vi "File handling.vi"(1 "Loop ID":u16, 11 "error out":errorcluster) -> ()   [LabVIEW 2011]
uses:
  Status Digitalish.ctl
  emi Lib/System 01/0 - General/App/Loop control 2/Private/_emi_ SMLoop start condition.vi
  emi Lib/System 01/0 - General/App/Loop control 2/Private/_emi_ SMLoop Error Check.vi
  emi Lib/Basic/0 - General/Error/emi_Is Error.vi
  emi Lib/System 01/0 - General/App/Loop control 2/Private/_emi_SMLoop Register new.vi
  emi Lib/System 01/0 - General/S&E reporting/emi_Send S&E Error message.vi
  emi Lib/Basic/0 - General/Error/emi_ Is Error state.vi
  emi Lib/System 01/0 - General/emi_Read System ID.vi
  emi Lib/System 01/0 - General/App/Loop control/Private/_emi_GFV Loop Linking.vi
  emi Lib/System 01/0 - General/App/Loop control/Private/_emi_GFV Loop Enable.vi
  emi Lib/System 01/0 - General/App/Loop control 2/Private/_emi_ SMLoop Restart.vi
  emi Lib/System 01/0 - General/App/Private/_emi_GFV App Close.vi
  emi Lib/System 01/0 - General/App/Loop control 2/Private/_emi_ SMLoop Restart Counter.vi
  emi Lib/System 01/0 - General/App/Loop control/Private/_emi_GFV Loop Running.vi
  emi Lib/System 01/0 - General/Private/_emi_GFV System ID.vi
  emi Lib/System 01/0 - General/S&E reporting/Private/_emi_S&E Q Generator.vi
  emi Lib/System 01/0 - General/App/Loop control/Private/_emi_GFV stop a loop so it can reset.vi
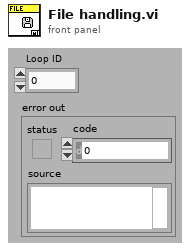
[diagram p1: front panel]
types:
  T1 = typedef "Status Digitalish.ctl" = enum16{"NA", "False", "True"}
  T2 = enum16{"open", "replace", "create", "open or create", "replace or create", "replace or create with confirmation"}
  T3 = typedef "_emi_ SMLoop sates.ctl" = enum16{"Init", "Standby", "Start", "Normal Operation", "Stop", "Error Handling", "End", "Post"}
  T4 = cluster{"Placeholder":bool, "ASCII log file":refnum<file>, "Bin log file":refnum<file>, "Analog Data":dbl[], "Digital Data":T1[]}
  T5 = typedef "Ch Info dbl.ctl" = cluster{"Name":string, "Unit":string, "Aditional":i32}
  T6 = typedef "Ch Info u8 std.ctl" = cluster{"Name":string, "Aditional":i32}
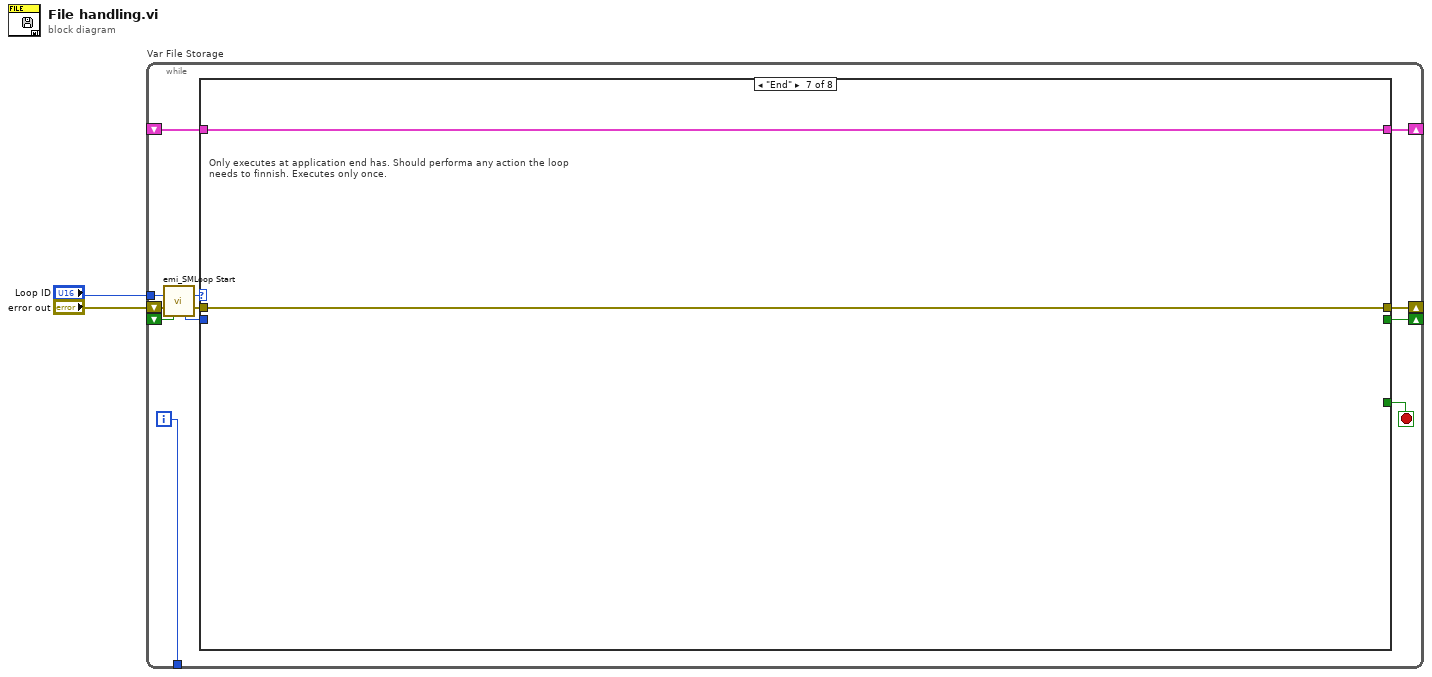
[diagram p0: block diagram]
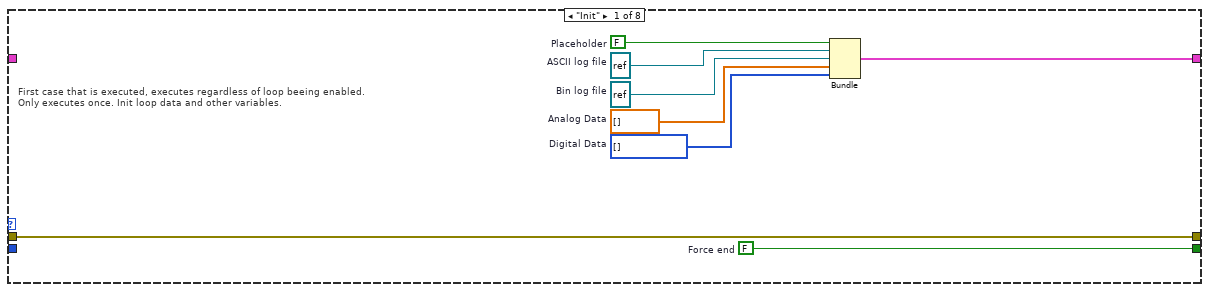
[diagram p2: hidden frame]
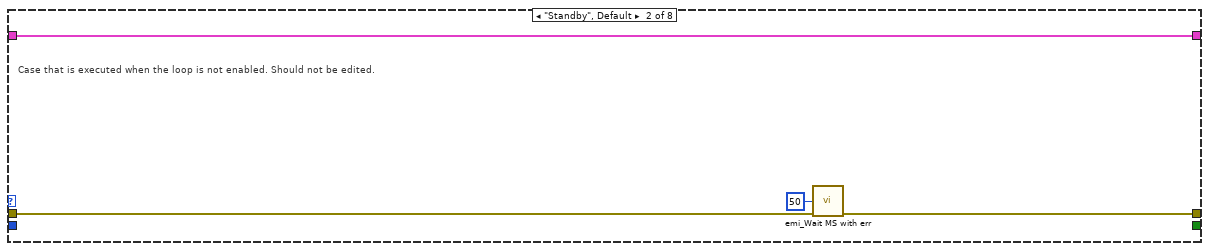
[diagram p3: hidden frame]
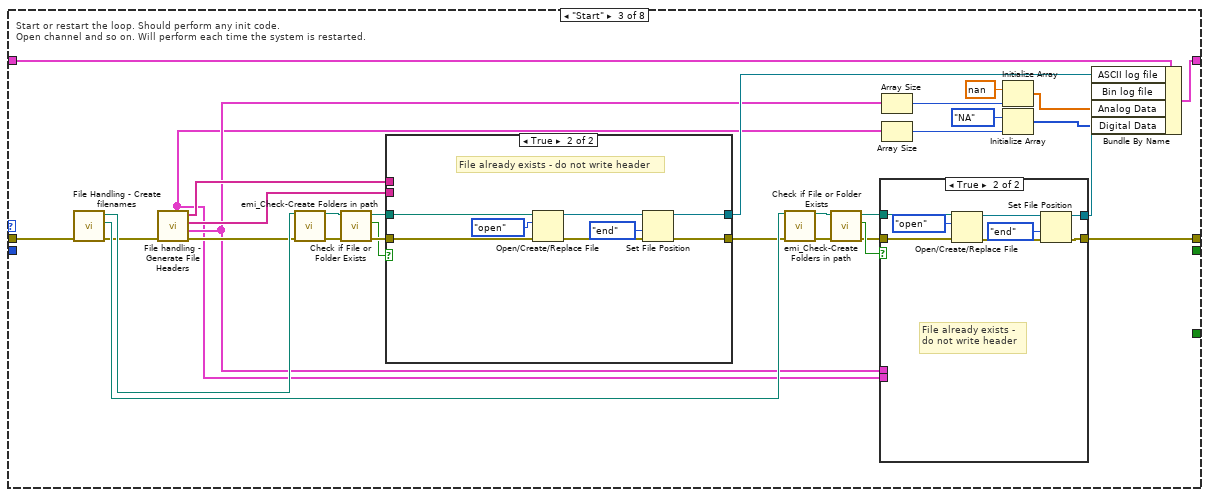
[diagram p4: hidden frame]
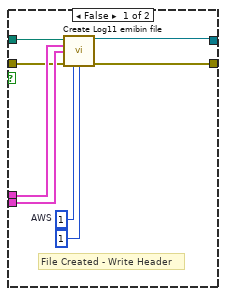
[diagram p5: hidden frame]
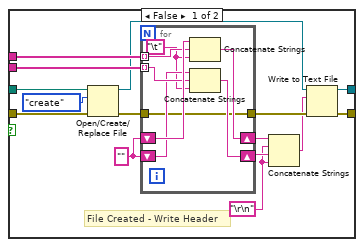
[diagram p6: hidden frame]
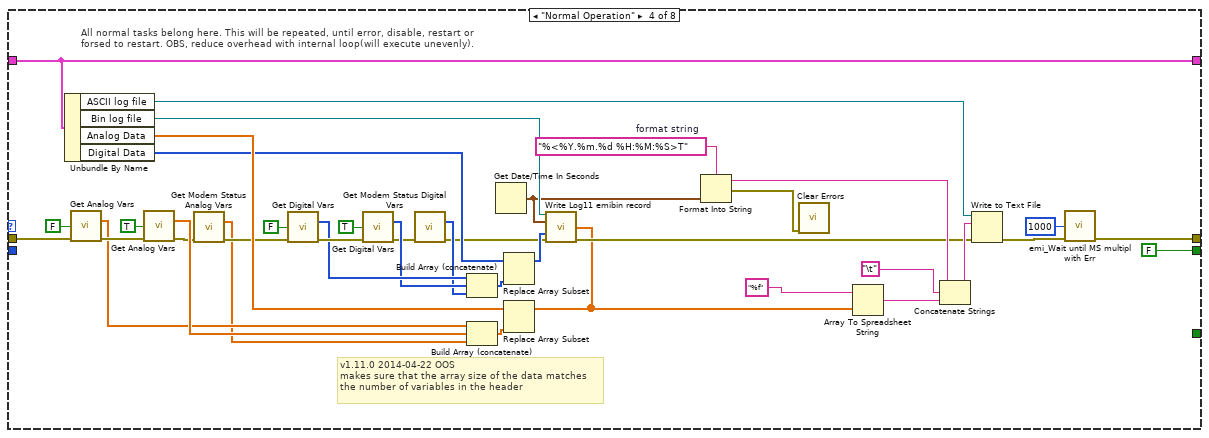
[diagram p7: hidden frame]
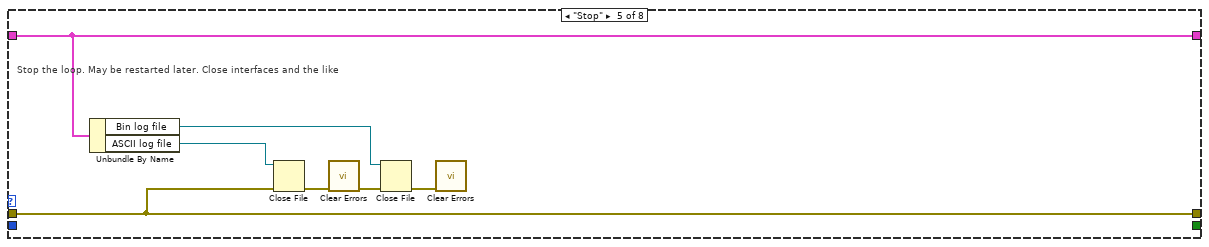
[diagram p8: hidden frame]
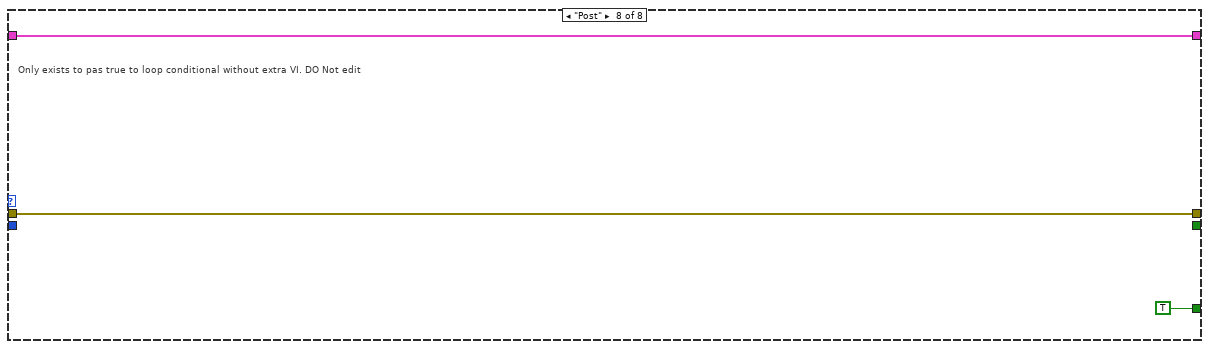
[diagram p10: hidden frame]
diagram:
  n1 = while "Var File Storage" {
    shift-right: [w14] -> _
    shift-left: _ -> [w10]
    shift-right: [w12] -> _
    shift-left: "error out" -> [w8]
    tunnel: [w11] -> _
    shift-right: [w9] -> _
    shift-left: _ -> [w4]
    tunnel: "Loop ID" -> [w5]
    i -> [w11]
    stop <- w13 stop-if-true
    n2 = call "emi_SMLoop Start.vi"("Loop ID"=w5, "error in (no error)"=w8, "Force Stop(F)"=w4) -> ("Loop command"=w6:T3, "error out"=w7:errorcluster, "Loop ID out"=w3:i32)  [unwired: 10 in]
    n3 = case shown="\"End\"" w6 {
      tunnel: [w21 w23 w56 w141 w150 w152 w153 w156] -> w14
      tunnel: [_ _ _ _ _ _ _ TRUE] -> w13
      tunnel: w7 -> [w22 w25 w39 w143 w148 w151 w154 w157]
      tunnel: [w22 w24 w37 w142 w148 w151 w154 w157] -> w12
      tunnel: w10 -> [_ w23 w57 w141 w150 w152 w153 w156]
      tunnel: [w19 _ _ FALSE ("Force End") _ _ _ _] -> w9
      tunnel: w3 -> [_ _ _ _ _ _ _ _]
      frame "Init" {
        w15 = T1[] [] items=["NA", "False", "True"]  # Digital Data
        w16 = dbl[] []  # Analog Data
        w17 = refnum<file> refnum  # Bin log file
        w18 = refnum<file> refnum  # ASCII log file
        w19 = FALSE  # Force end
        w20 = FALSE  # Placeholder
        # "First case that is executed, executes regardless of loop beeing enabled.\nOnly executes once. Init loop data and other variables."
        n4 = Bundle("Placeholder"=w20, "ASCII log file"=w18, "Bin log file"=w17, "Analog Data"=w16, "Digital Data"=w15) -> (w21:T4)  [unwired: 1 in]
      }
      frame "Standby", Default {
        # "Case that is executed when the loop is not enabled. Should not be edited."
        n5 = call "emi_Wait MS with err.vi"("milliseconds to wait(0)"=u32 50, "error in (no error)"=w25) -> ("error out"=w24:errorcluster)  [unwired: 13 in]
      }
      frame "Start" {
        # "Start or restart the loop. Should perform any init code. \nOpen channel and so on. Will perform each time the system is restarted."
        n6 = call "File Handling - Create filenames.vi"("error in"=w39) -> ("error out"=w40:errorcluster, "Binary Logfile path"=w50:path, "ASCII Logfile path"=w55:path)  [unwired: 7 in, 1 out]
        n7 = call "File handling - Generate File Headers.vi"("error in (no error)"=w40) -> ("error out"=w51:errorcluster, "Analog Variables"=w48:T5[], "Column Units"=w53:string[], "Column Names"=w54:string[], "Digital Variables"=w47:T6[])  [unwired: 6 in]
        n8 = call "emi_Check-Create Folders in path.vi"("Path including file"=w55, "error in (no error)"=w51) -> ("Path out"=w36:path, "error out"=w35:errorcluster)  [unwired: 11 in, 1 out]
        n9 = call <vilib>:"Check if File or Folder Exists.vi"("error in (no error)"=w35, "path"=w36) -> ("error out"=w33:errorcluster, "file or folder exists?"=w32:bool, "dup path"=w34:path)  [unwired: 7 in]
        n10 = case shown="True" w32 {
          tunnel: w54 -> [w88 _]
          tunnel: w53 -> [w87 _]
          tunnel: [w80 w99] -> w52
          tunnel: [w76 w98] -> w38
          tunnel: w34 -> [w75 w103]
          tunnel: w33 -> [w74 w102]
          frame False {
            w83 = "\r\n"
            w86 = ""
            # "File Created - Write Header"
            n11 = Open/Create/Replace File(file path (use dialog)=w75, error in=w74, operation (0:open)=T2."create") -> (refnum out=w79:refnum<file>, error out=w77:errorcluster)  [unwired: 3 in, 1 out]
            n12 = for {
              tunnel: w77 -> [w90]
              tunnel: w88 -> [w95] mode=indexing
              tunnel: w87 -> [w93] mode=indexing
              shift-right: [w94] -> w85
              shift-left: w86 -> [w96]
              shift-right: [w91] -> w84
              shift-left: w86 -> [w92]
              tunnel: [w90] -> w82
              w89 = "\t"
              n13 = Concatenate Strings(w96, w95, w89) -> (w94:string)
              n14 = Concatenate Strings(w92, w93, w89) -> (w91:string)
            }
            n15 = Concatenate Strings(w85, w83, w84, w83) -> (w81:string)
            n16 = Write to Text File(file (use dialog)=w79, text=w81, error in=w82) -> (refnum out=w80:refnum<file>, error out=w76:errorcluster)  [unwired: 1 in, 1 out]
          }
          frame True {
            # "File already exists - do not write header"
            n17 = Open/Create/Replace File(file path (use dialog)=w103, error in=w102, operation (0:open)=T2."open") -> (refnum out=w101:refnum<file>, error out=w100:errorcluster)  [unwired: 3 in, 1 out]
            n18 = Set File Position(refnum=w101, from (0:start)=enum16{"start", "end", "current"}."end", error in=w100) -> (refnum out=w99:refnum<file>, error out=w98:errorcluster)  [unwired: 1 in]
          }
        }
        n19 = call "emi_Check-Create Folders in path.vi"("Path including file"=w50, "error in (no error)"=w38) -> ("Path out"=w31:path, "error out"=w30:errorcluster)  [unwired: 11 in, 1 out]
        n20 = call <vilib>:"Check if File or Folder Exists.vi"("error in (no error)"=w30, "path"=w31) -> ("error out"=w28:errorcluster, "file or folder exists?"=w29:bool, "dup path"=w27:path)  [unwired: 7 in]
        n21 = case shown="True" w29 {
          tunnel: [w63 w67] -> w49
          tunnel: w48 -> [w62 _]
          tunnel: w47 -> [w61 _]
          tunnel: [w60 w66] -> w37
          tunnel: w28 -> [w59 w73]
          tunnel: w27 -> [w58 w72]
          frame False {
            w65 = u16 1  # AWS
            # "File Created - Write Header"
            n22 = call "Create Log11 emibin file.vi"("file path"=w58, "dbl Array"=w62, "u8 std Array"=w61, "error in"=w59, "File type ID(0, generic)"=w65, "File type Version(0, Unset)"=u8 1) -> ("refnum out"=w63:refnum<file>, "error out"=w60:errorcluster)  [unwired: 8 in]
          }
          frame True {
            # "File already exists - \ndo not write header"
            n23 = Open/Create/Replace File(file path (use dialog)=w72, error in=w73, operation (0:open)=T2."open") -> (refnum out=w69:refnum<file>, error out=w68:errorcluster)  [unwired: 3 in, 1 out]
            n24 = Set File Position(refnum=w69, from (0:start)=enum16{"start", "end", "current"}."end", error in=w68) -> (refnum out=w67:refnum<file>, error out=w66:errorcluster)  [unwired: 1 in]
          }
        }
        n25 = Array Size(array=w48) -> (size(s)=w46:i32)
        n26 = Array Size(array=w47) -> (size(s)=w43:i32)
        n27 = Initialize Array(nan ("element"), w46) -> (w45:dbl[])
        n28 = Initialize Array(Status_Digitalish."NA", w43) -> (w41:T1[])
        n29 = Bundle By Name(cluster=w57, "ASCII log file"=w52, "Bin log file"=w49, "Analog Data"=w45, "Digital Data"=w41) -> (w56:T4)
      }
      frame "Normal Operation" {
        w122 = "%<%Y.%m.%d %H:%M:%S>T"  # format string
        # "v1.11.0 2014-04-22 OOS\nmakes sure that the array size of the data matches\nthe number of variables in the header"
        # "All normal tasks belong here. This will be repeated, until error, disable, restart or\nforsed to restart. OBS, reduce overhead with internal loop(will execute unevenly)."
        n30 = Unbundle By Name(w141) -> ("ASCII log file"=w138:refnum<file>, "Bin log file"=w124:refnum<file>, "Analog Data"=w116:dbl[], "Digital Data"=w113:T1[])
        n31 = call "Get Analog Vars.vi"("Tool"=FALSE, "error in (no error)"=w143) -> ("Values"=w119:dbl[], "error out"=w134:errorcluster)  [unwired: 7 in, 5 out]
        n32 = call "Get Analog Vars.vi"("Tool"=TRUE, "error in (no error)"=w134) -> ("Values"=w120:dbl[], "error out"=w107:errorcluster)  [unwired: 7 in, 5 out]
        n33 = call "Get Modem Status Analog Vars.vi"("error in (no error)"=w107) -> ("Values"=w105:dbl[], "error out"=w106:errorcluster)  [unwired: 8 in, 5 out]
        n34 = call "Get Digital Vars.vi"("Tool"=FALSE, "error in (no error)"=w106) -> ("Values"=w118:T1[], "error out"=w127:errorcluster)  [unwired: 7 in, 5 out]
        n35 = call "Get Digital Vars.vi"("Tool"=TRUE, "error in (no error)"=w127) -> ("Values"=w117:T1[], "error out"=w110:errorcluster)  [unwired: 7 in, 5 out]
        n36 = call "Get Modem Status Digital Vars.vi"("error in (no error)"=w110) -> ("Values"=w109:T1[], "error out"=w108:errorcluster)  [unwired: 8 in, 5 out]
        n37 = Build Array (concatenate)(w118, w117, w109) -> (w112:T1[])
        n38 = Build Array (concatenate)(w119, w120, w105) -> (w115:dbl[])
        n39 = Get Date/Time In Seconds() -> (seconds since 1Jan1904=w123:timestamp)
        n40 = Replace Array Subset(array=w113, new element=w112) -> (w111:T1[])  [unwired: 1 in]
        n41 = Replace Array Subset(array=w116, new element=w115) -> (w114:dbl[])  [unwired: 1 in]
        n42 = call "Write Log11 emibin record.vi"("refnum in"=w124, "Time"=w123, "Doubles"=w114, "u8"=w111, "error in"=w108) -> ("error out"=w125:errorcluster)  [unwired: 9 in, 1 out]
        n43 = Format Into String(format string=w122, w123) -> (resulting string=w129:string, error out=w121:errorcluster)  [unwired: 2 in]
        n44 = call <vilib>:"Clear Errors.vi"("error in (no error)"=w121) -> ()  [unwired: 6 in, 1 out]
        n45 = Array To Spreadsheet String(array=w114, 3:"%f" ("format string")) -> (spreadsheet string=w132:string)  [unwired: 1 in]
        n46 = Concatenate Strings(w129, "\t", w132) -> (w131:string)
        n47 = Write to Text File(file (use dialog)=w138, text=w131, error in=w125) -> (error out=w137:errorcluster)  [unwired: 1 in, 2 out]
        n48 = call "emi_Wait until MS multipl with Err.vi"("millisecond multiple(0)"=u32 1000 ("milliseconds to wait(0)"), "error in (no error)"=w137) -> ("error out"=w142:errorcluster)  [unwired: 13 in]
      }
      frame "Stop" {
        # "Stop the loop. May be restarted later. Close interfaces and the like"
        n49 = Unbundle By Name(w150) -> ("Bin log file"=w144:refnum<file>, "ASCII log file"=w149:refnum<file>)
        n50 = Close File(refnum=w149, error in=w148) -> (error out=w147:errorcluster)  [unwired: 1 out]
        n51 = call <vilib>:"Clear Errors.vi"("error in (no error)"=w147) -> ("error out"=w145:errorcluster)  [unwired: 6 in]
        n52 = Close File(refnum=w144, error in=w145) -> (error out=w146:errorcluster)  [unwired: 1 out]
        n53 = call <vilib>:"Clear Errors.vi"("error in (no error)"=w146) -> ()  [unwired: 6 in, 1 out]
      }
      frame "Error Handling" {
        # "Loop automaticaly returns here after error is found. If error is cleared, \nLoop wil continue as normal(if was operative when error."
      }
      frame "End" {
        # "Only executes at application end has. Should performa any action the loop \nneeds to finnish. Executes only once."
      }
      frame "Post" {
        # "Only exists to pas true to loop conditional without extra VI. DO Not edit"
      }
    }
  }
